vi "Configure VNA 2 Port Meas.vi"(0 "Semiconductor Module Context":T2, 5 "Calibration File Paths":path[](array[path]), 9 "Pins":string[](array[string]), 11 "error in (no error)":errorcluster) -> (4 "VNA Calibration Parameters":T1, 15 "error out":errorcluster)   [LabVIEW 2013]
uses:
  <vilib>/NI_TestStand_SemiconductorModule/NI_TestStand_Semiconductor_Module.lvlibp/PinMap/General/SemiconductorModuleContext.ctl
  VNA Calibration Parameters.ctl
  <vilib>/NI_TestStand_SemiconductorModule/NI_TestStand_Semiconductor_Module.lvlibp/PinMap/General/NIInstrumentTypeIDs.ctl
  <instrlib>/niVNA/niVNA.llb/niVNA Load Calibration And Configuration Data From File.vi
  Pin Map API/VNA Custom Instrument.lvlib
  <vilib>/NI_TestStand_SemiconductorModule/NI_TestStand_Semiconductor_Module.lvlibp
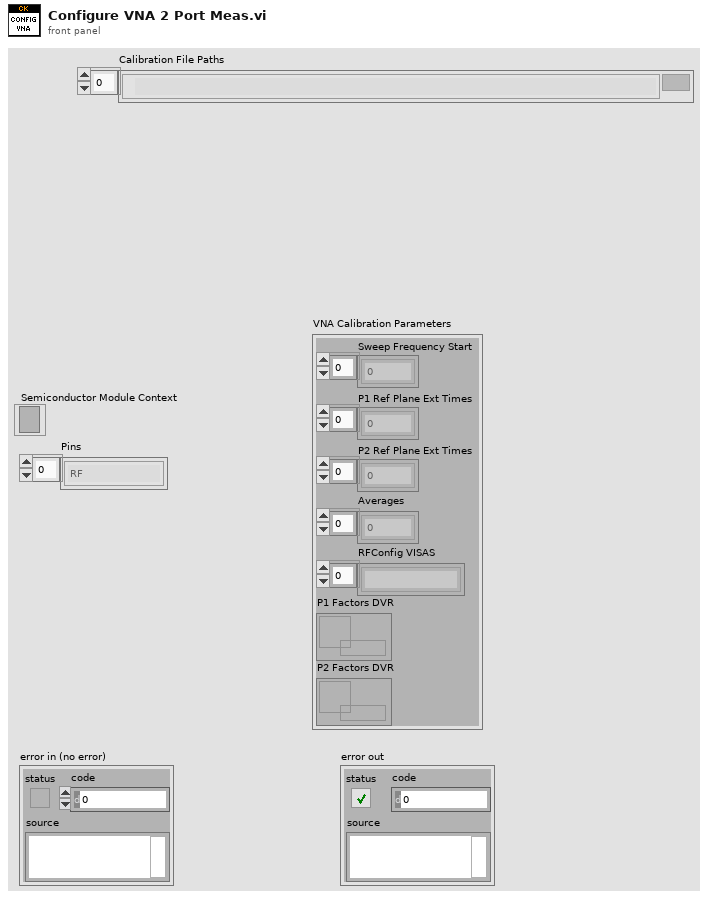
[diagram p1: front panel]
types:
  T1 = typedef "VNA Calibration Parameters.ctl" = cluster{"Sweep Frequency Start":dbl[], "P1 Ref Plane Ext Times":dbl[], "P2 Ref Plane Ext Times":dbl[], "Averages":i32[], "RFConfig VISAS":string[], "P1 Factors DVR":refnum<data-value>, "P2 Factors DVR":refnum<data-value>}
  T2 = typedef "NI_TestStand_Semiconductor_Module.lvlibp/SemiconductorModuleContext.ctl" = refnum<k7>
  T3 = typedef "NI_TestStand_Semiconductor_Module.lvlibp/NIInstrumentTypeIDs.ctl" = string
  T4 = typedef "Two Port Corerction Factors.ctl" = cluster{"Forward e00":cdb[], "Forward e11":cdb[], "Forward e10e01":cdb[], "Forward e30":cdb[], "Forward e22":cdb[], "Forward e10e32":cdb[], "Reverse e33":cdb[], "Reverse e22 ":cdb[], "Reverse e23e32":cdb[], "Reverse e03":cdb[], "Reverse e11":cdb[], "Reverse e23e01":cdb[]}
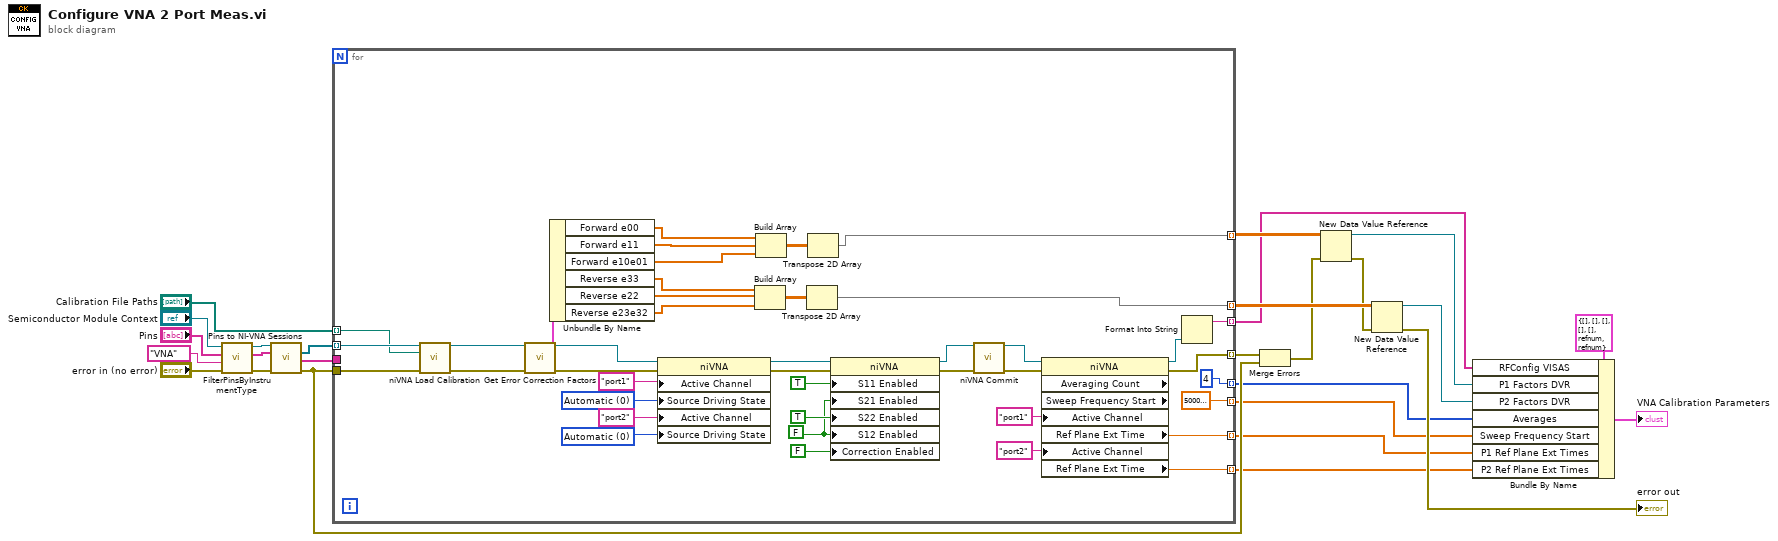
[diagram p0: block diagram]
diagram:
  n1 = call <vilib>:"FilterPinsByInstrumentType.vi"("error in (no error)"="error in (no error)", "Instrument Type Id"=T3 "VNA", "Pins"="Pins", "Semiconductor Module Context"="Semiconductor Module Context") -> ("error out"=w24:errorcluster, "Filtered Pins"=w23:string[], "Semiconductor Module Context Out"=w22:T2)  [unwired: 5 in]
  n2 = call "Pins to NI-VNA Sessions.vi"("Semiconductor Module Context"=w22, "Pins"=w23, "error in (no error)"=w24) -> ("Instrument Sessions"=w26:refnum<k15>[], "Channel Lists"=w25:string[], "error out"=w10:errorcluster)  [unwired: 8 in, 2 out]
  n3 = for {
    tunnel: w26 -> [w66] mode=indexing
    tunnel: "Calibration File Paths" -> [w65] mode=indexing
    tunnel: w25 -> [_]
    tunnel: [50000000.0 ("Sweep Frequency Start")] -> w3 mode=indexing
    tunnel: [w44] -> w18 mode=indexing
    tunnel: [w43] -> w17 mode=indexing
    tunnel: w10 -> [w67]
    tunnel: [w64] -> w11 mode=indexing
    tunnel: [w40] -> w2 mode=indexing
    tunnel: [w39] -> w1 mode=indexing
    tunnel: [4 ("Averaging Count")] -> w4 mode=indexing
    tunnel: [w36] -> w7 mode=indexing
    w35 = FALSE ("Calibration Settings:Correction Enabled")
    w49 = 0 items=["Automatic", "Active", "Inactive"] ("Individual Sources/Receiver:Source Driving State")
    w59 = 0 items=["Automatic", "Active", "Inactive"] ("Individual Sources/Receiver:Source Driving State")
    n4 = call-poly <instrlib>:"niVNA Load Calibration.vi"("instrument handle"=w66, "file path"=w65, "error in"=w67) -> ("instrument handle out"=w62:refnum<k15>, "error out"=w61:errorcluster)  [unwired: 11 in]
    n5 = call "Get Error Correction Factors.vi"("instrument handle"=w62, "Error In"=w61) -> ("instrument handle out"=w51:refnum<k15>, "Two Port Correction Factors"=w45:T4, "Error Out"=w52:errorcluster)  [unwired: 11 in]
    n6 = Unbundle By Name(w45) -> ("Forward e00"=w33:cdb[], "Forward e11"=w32:cdb[], "Forward e10e01"=w31:cdb[], "Reverse e33"=w30:cdb[], "Reverse e22"=w29:cdb[], "Reverse e23e32"=w28:cdb[])
    n7 = property class="niVNA"(reference=w51, error in=w52, "Active Channel"="port1", "Source Driving State"=w59, "Active Channel"="port2", "Source Driving State"=w49) -> (reference out=w56:refnum<k15>, error out=w57:errorcluster)
    n8 = Build Array(w30, w29, w28) -> (w46:cdb[][])
    n9 = Build Array(w33, w32, w31) -> (w47:cdb[][])
    n10 = Transpose 2D Array(2D array=w46) -> (transposed array=w43:cdb[][])
    n11 = Transpose 2D Array(2D array=w47) -> (transposed array=w44:cdb[][])
    n12 = property class="niVNA"(reference=w56, error in=w57, "S11 Enabled"=TRUE ("Sweep:S11 Enabled"), "S21 Enabled"=w35, "S22 Enabled"=TRUE ("Sweep:S11 Enabled"), "S12 Enabled"=w35, "Correction Enabled"=FALSE ("Calibration Settings:Correction Enabled")) -> (reference out=w50:refnum<k15>, error out=w48:errorcluster)
    n13 = call <instrlib>:"niVNA Commit.vi"("instrument handle"=w50, "error in"=w48) -> ("instrument handle out"=w38:refnum<k15>, "error out"=w63:errorcluster)  [unwired: 12 in]
    n14 = property class="niVNA" props=["Averaging Count", "Sweep Frequency Start", "Active Channel", "Ref Plane Ext Time", "Active Channel", "Ref Plane Ext Time"](reference=w38, error in=w63, "Active Channel"="port1", "Active Channel"="port2") -> (reference out=w37:refnum<k15>, error out=w64:errorcluster, "Ref Plane Ext Time"=w40:dbl, "Ref Plane Ext Time"=w39:dbl)  [unwired: 2 out]
    n15 = Format Into String(w37) -> (resulting string=w36:string)  [unwired: 3 in, 1 out]
  }
  n16 = Merge Errors(w11, w10) -> (w12:errorcluster)
  n17 = New Data Value Reference(data value=w18, error in=w12) -> (data value reference=w6:refnum<data-value>, error out=w16:errorcluster)
  n18 = New Data Value Reference(data value=w17, error in=w16) -> (data value reference=w5:refnum<data-value>, error out=→"error out":errorcluster)
  n19 = Bundle By Name(cluster=T1 {"Sweep Frequency Start"=[], "P1 Ref Plane Ext Times"=[], "P2 Ref Plane Ext Times"=[], "Averages"=[], "RFConfig VISAS"=[], "P1 Factors DVR"=refnum, "P2 Factors DVR"=refnum} ("VNA Measurement Parameters 2"), "RFConfig VISAS"=w7, "P1 Factors DVR"=w6, "P2 Factors DVR"=w5, "Averages"=w4, "Sweep Frequency Start"=w3, "P1 Ref Plane Ext Times"=w2, "P2 Ref Plane Ext Times"=w1) -> (→"VNA Calibration Parameters":T1)
